vi "1D kinematics step.vi"(0 "time step (s)":dbl=0.01, 7 "starting state":T1={"position (m)"=5.0, "velocity (m/s)"=10.0}, 11 "acceleration(m/s^2)":dbl=9.8) -> (8 "ending state":T1={"position (m)"=5.0, "velocity (m/s)"=10.0})   [LabVIEW 2016]
doc: "This subvi updates the 1D velocity and position of an object given the acceleration and a small time step.\n\nPaul K Dixon\nP350\nCSUSB Physics"
uses:
  typedef/1d state.ctl
panel:
  # "Kinematics update in 1D"
  # "update parameters"
  # "Paul K Dixon\nP350"
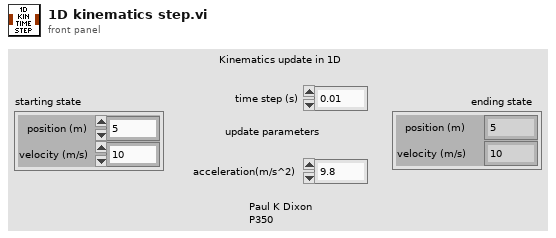
[diagram p1: front panel]
types:
  T1 = typedef "1d state.ctl" = cluster{"position (m)":dbl, "velocity (m/s)":dbl}
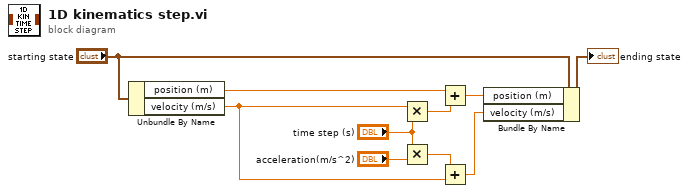
[diagram p0: block diagram]
diagram:
  n1 = Unbundle By Name("starting state") -> ("position (m)"=w6:dbl, "velocity (m/s)"=w1:dbl)
  n2 = Multiply(x=w1, y="time step (s)") -> (x*y=w7:dbl)
  n3 = Multiply(x="time step (s)", y="acceleration(m/s^2)") -> (x*y=w9:dbl)
  n4 = Add(x=w6, y=w7) -> (x+y=w5:dbl)
  n5 = Add(x=w9, y=w1) -> (x+y=w2:dbl)
  n6 = Bundle By Name(cluster="starting state", "position (m)"=w5, "velocity (m/s)"=w2) -> (→"ending state":T1)
